vi "onProcessStart.vi"(8 "error in (no error)":errorcluster, 11 "DAQmx-AI":refnum<class "DAQmx-AI.lvclass">) -> (0 "error out":errorcluster, 3 "DAQmx-AI out":refnum<class "DAQmx-AI.lvclass">)   [LabVIEW 2016, in "DAQmx-AI.lvclass"]
doc: "JKI State Machine Objects (SMO) 1.1.8.32\nJKI - JKI\nCopyright (c) 2016, JKI"
uses:
  DAQmx-AI.lvclass
  <vilib>/DAQmx/create/channels.llb/DAQmx Create Channel (AI-Voltage-Basic).vi
  <vilib>/DAQmx/create/channels.llb/DAQmx Create Channel (AI-Current-Basic).vi
  <vilib>/DAQmx/configure/task.llb/DAQmx Configure Logging (TDMS).vi
  <vilib>/JKI/JKI SMO/SMO/SMO.lvclass
  <resource>/objmgr/daqmx.rc
panel:
  # "For instructions on how to use the JKI State Machine Objects, examples and video tutorials, visit:\nhttp://jki.net/state-machine-objects/\n\nJKI State Machine Objects™\nhttp://jki.net/state-machine-objects/\nCopyright (C) 2005-2015, JKI <info@jki.net>\nALL RIGHTS RESERVED"
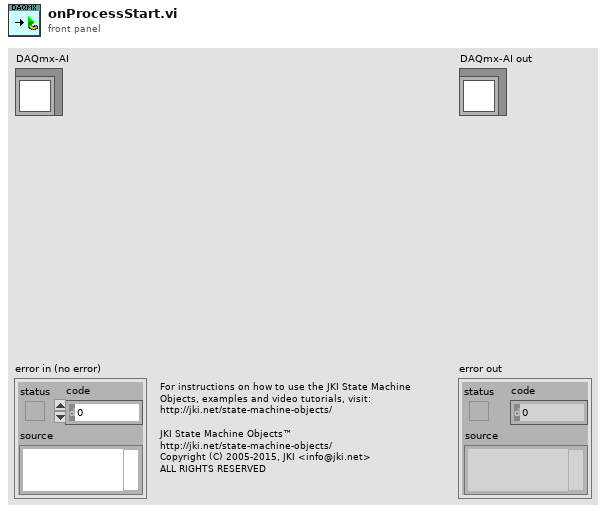
[diagram p1: front panel]
types:
  T1 = typedef "DAQmx-AI.lvclass/Configuration--Cluster.ctl" = cluster{"PhysChan":tag, "Period (ms)":i64, "input terminal cfg":i32, "minimum value":dbl, "maximum value":dbl, "units":T2, "task name":string, "TDMS File Path":path, "Group Name":string}
  T2 = typedef "DAQmx-AI.lvclass/Units -- Enum.ctl" = enum16{"Volts", "Amps", "Deg F", "Deg C", "Deg R", "Kelvins", "Strain", "Ohms", "Hz", "Seconds", "Meters", "Inches", "Degrees", "Radians", "Ticks", "g", "m/s^2", "m/s", "in/s", "Pascals", "Newtons", "Pounds", "kgf", "psi", "bar", "Nm", "oz-in", "lb-in", "lb-ft", "Volts/Volt", "mVolts/Volt", "From TEDS"}
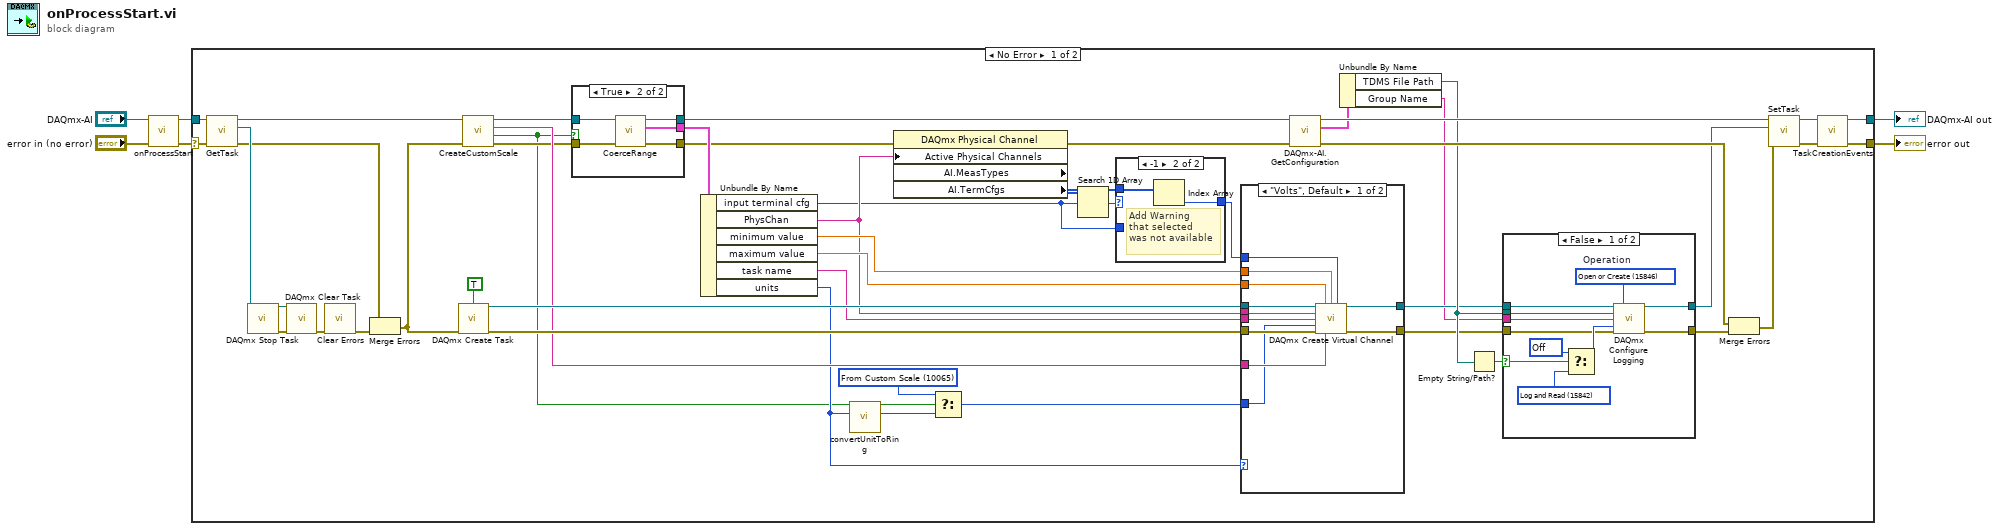
[diagram p0: block diagram]
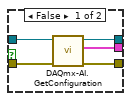
[diagram p4: hidden frame]
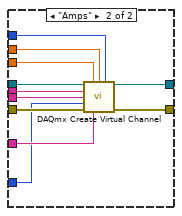
[diagram p5: hidden frame]
diagram:
  n1 = call-parent "onProcessStart.vi"("error in (no error)"="error in (no error)", "SMO"="DAQmx-AI") -> ("error out"=w1:errorcluster, "SMO out"=w4:refnum<class "DAQmx-AI.lvclass">)  [unwired: 8 in]
  n2 = case shown="No Error" w1 {
    selector: w1 -> [w49 w104]
    tunnel: w4 -> [w50 w103]
    tunnel: [w19 w103] -> w3
    tunnel: [w20 w104] -> w2
    frame No Error {
      w32 = 10065 items=["Volts"=10348, "From Custom Scale"=10065] ("units")
      n3 = call "GetTask.vi"("error in (no error)"=w49, "DAQmx-AI"=w50) -> ("error out"=w43:errorcluster, "task"=w46:refnum<k21>, "DAQmx-AI out"=w36:refnum<class "DAQmx-AI.lvclass">)  [unwired: 7 in]
      n4 = call <vilib>:"DAQmx Stop Task.vi"("task/channels in"=w46) -> ("task out"=w47:refnum<k21>, "error out"=w48:errorcluster)  [unwired: 13 in]
      n5 = call <vilib>:"DAQmx Clear Task.vi"("task in"=w47, "error in"=w48) -> ("error out"=w45:errorcluster)  [unwired: 13 in]
      n6 = call <vilib>:"Clear Errors.vi"("error in (no error)"=w45) -> ("error out"=w44:errorcluster)  [unwired: 5 in, 1 out]
      n7 = Merge Errors(w43, w44) -> (w35:errorcluster)
      n8 = call <vilib>:"DAQmx Create Task.vi"("auto cleanup"=TRUE, "error in"=w35) -> ("task out"=w54:refnum<k21>, "error out"=w53:errorcluster)  [unwired: 12 in]
      n9 = call "CreateCustomScale.vi"("error in (no error)"=w35, "DAQmx-AI"=w36) -> ("error out"=w28:errorcluster, "Custom Scaling"=w27:bool, "Custom Scale"=w34:tag, "DAQmx-AI out"=w29:refnum<class "DAQmx-AI.lvclass">)  [unwired: 6 in]
      n10 = case shown="True" w27 {
        tunnel: [w71 w76] -> w52
        tunnel: [w72 w80] -> w17
        tunnel: [w73 w79] -> w25
        tunnel: w29 -> [w75 w78]
        tunnel: w28 -> [w74 w77]
        frame False {
          n11 = call "DAQmx-AI.GetConfiguration.vi"("error in (no error)"=w74, "DAQmx-AI"=w75) -> ("error out"=w73:errorcluster, "Configuration"=w71:T1, "DAQmx-AI out"=w72:refnum<class "DAQmx-AI.lvclass">)  [unwired: 7 in]
        }
        frame True {
          n12 = call "CoerceRange.vi"("error in (no error)"=w77, "DAQmx-AI"=w78) -> ("error out"=w79:errorcluster, "Configuration"=w76:T1, "DAQmx-AI out"=w80:refnum<class "DAQmx-AI.lvclass">)  [unwired: 7 in]
        }
      }
      n13 = Unbundle By Name(w52) -> ("input terminal cfg"=w21:i32, "PhysChan"=w26:tag, "minimum value"=w39:dbl, "maximum value"=w38:dbl, "task name"=w37:string, "units"=w33:T2)
      n14 = call "convertUnitToRing.vi"("Units"=w33) -> ("DAQmx units (Ring)"=w31:i32)  [unwired: 10 in]
      n15 = property class="DAQmx Physical Channel" props=["Active Physical Channels", "AI.MeasTypes", "AI.TermCfgs"](error in=w25, "Active Physical Channels"=w26) -> (error out=w16:errorcluster, "AI.TermCfgs"=w23:i32[])  [unwired: 1 in, 2 out]
      n16 = Select(t=w32, s=w27, f=w31) -> (s? t:f=w30:i32)
      n17 = Search 1D Array(1D array=w23, element=w21) -> (index of element=w24:i32)  [unwired: 1 in]
      n18 = case shown="-1" w24 {
        tunnel: w23 -> [_ w70]
        tunnel: [w68 w69] -> w22
        tunnel: w21 -> [w68 _]
        frame Default {
        }
        frame -1 {
          # "Add Warning\nthat selected\nwas not available"
          n19 = Index Array(array=w70) -> (element=w69:i32)  [unwired: 1 in]
        }
      }
      n20 = case shown="\"Volts\", Default" w33 {
        tunnel: w54 -> [w91 w102]
        tunnel: w53 -> [w90 w101]
        tunnel: w26 -> [w89 w100]
        tunnel: [w88 w99] -> w9
        tunnel: [w87 w98] -> w11
        tunnel: w22 -> [w86 w97]
        tunnel: w39 -> [w85 w96]
        tunnel: w38 -> [w84 w95]
        tunnel: w37 -> [w83 w94]
        tunnel: w34 -> [w82 w93]
        tunnel: w30 -> [w81 w92]
        frame "Volts", Default {
          n21 = call-poly <vilib>:"DAQmx Create Virtual Channel.vi"("task in"=w91, "maximum value"=w84, "minimum value"=w85, "input terminal configuration"=w86, "physical channels"=w89, "name to assign"=w83, "units"=w81, "error in"=w90, "custom scale name"=w82) -> ("task out"=w87:refnum<k21>, "error out"=w88:errorcluster)  [unwired: 5 in]
        }
        frame "Amps" {
          n22 = call-poly <vilib>:"DAQmx Create Virtual Channel.vi"("task in"=w102, "maximum value"=w95, "minimum value"=w96, "input terminal configuration"=w97, "physical channels"=w100, "name to assign"=w94, "units"=w92, "error in"=w101, "custom scale name"=w93) -> ("task out"=w98:refnum<k21>, "error out"=w99:errorcluster)  [unwired: 5 in]
        }
      }
      n23 = call "DAQmx-AI.GetConfiguration.vi"("error in (no error)"=w16, "DAQmx-AI"=w17) -> ("error out"=w15:errorcluster, "Configuration"=w14:T1, "DAQmx-AI out"=w18:refnum<class "DAQmx-AI.lvclass">)  [unwired: 7 in]
      n24 = Unbundle By Name(w14) -> ("TDMS File Path"=w13:path, "Group Name"=w8:string)
      n25 = Empty String/Path?(string/path=w13) -> (empty?=w7:bool)
      n26 = case shown="False" w7 {
        selector: w7 -> [w55 _]
        tunnel: w13 -> [w61 _]
        tunnel: [w60 w67] -> w12
        tunnel: w11 -> [w59 w67]
        tunnel: [w58 w66] -> w10
        tunnel: w9 -> [w57 w66]
        tunnel: w8 -> [w56 _]
        frame False {
          w62 = 10231 items=["Off"=10231, "Log"=15844, "Log and Read"=15842] ("logging mode")
          w64 = 15842 items=["Off"=10231, "Log"=15844, "Log and Read"=15842] ("logging mode")
          w65 = 15846 items=["Open"=10437, "Open or Create"=15846, "Create or Replace"=15847, "Create"=15848]  # Operation
          n27 = Select(t=w62, s=w55, f=w64) -> (s? t:f=w63:i32)
          n28 = call-poly <vilib>:"DAQmx Configure Logging.vi"("task/channels in"=w59, "operation"=w65, "file path"=w61, "group name"=w56, "logging mode"=w63, "error in"=w57) -> ("task out"=w60:refnum<k21>, "error out"=w58:errorcluster)  [unwired: 8 in]
        }
        frame True {
        }
      }
      n29 = Merge Errors(w15, w10) -> (w42:errorcluster)
      n30 = call "SetTask.vi"("error in (no error)"=w42, "task"=w12, "DAQmx-AI"=w18) -> ("error out"=w40:errorcluster, "DAQmx-AI out"=w41:refnum<class "DAQmx-AI.lvclass">)  [unwired: 7 in]
      n31 = call "TaskCreationEvents.vi"("error in (no error)"=w40, "DAQmx-AI"=w41) -> ("error out"=w20:errorcluster, "DAQmx-AI out"=w19:refnum<class "DAQmx-AI.lvclass">)  [unwired: 8 in]
    }
    frame Error {
    }
  }
  "error out" <- w2
  "DAQmx-AI out" <- w3
